vi "measure(SubVI).vi"(1 "config":refnum<queue>, 11 "error in (no error)":errorcluster) -> (4 "data":string[](array[string]), 15 "error out":errorcluster)   [LabVIEW 2019, in "SubVI.lvlib"]
uses:
  SubVI.lvlib
  config.ctl
  Instrument.ctl
  lib/QDInstrument.dll
  <vilib>/NI/Modbus Library/API/Master/Modbus Master.lvclass
  lib/Keithley 2400/Keithley 24XX/Public/Data/Read (Single Point).vi
  lib/Keithley 2400/Keithley 24XX/Keithley 24XX.lvlib
  <vilib>/measure/NI_MABase.lvlib
panel:
  # "(真是通道1，假是通道2)"
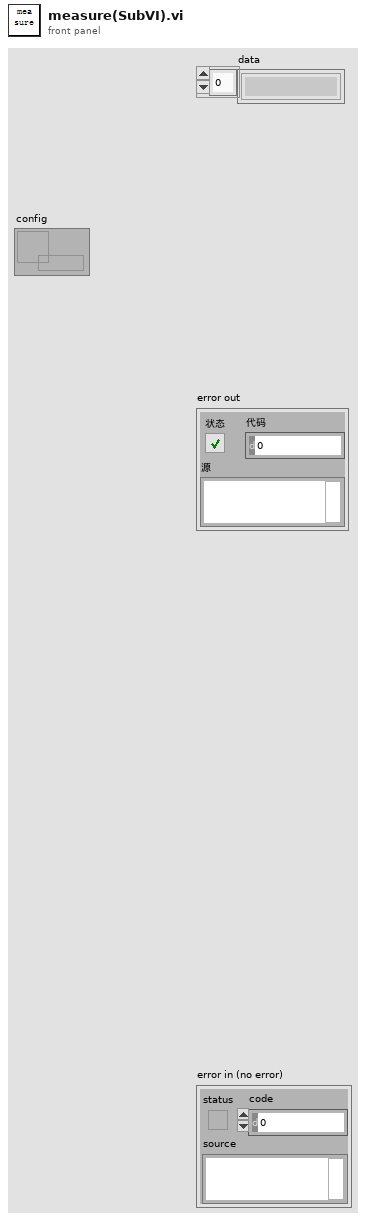
[diagram p1: front panel]
types:
  T1 = typedef "config.ctl" = cluster{"initialize":string, "6221":cluster{"6221 Resource":refnum<visa-resource-name>, "Delta status":bool}, "7001":cluster{"Ch":bool}, "SR830+6221":cluster{"source":u16, "阻抗":dbl, "量程入 4":i32, "量程入 3":i32, "量程入 2":i32, "量程入 1":i32, "电流":dbl, "SR830 2":bool, "SR830 3":bool, "SR830 4":bool, "SR830 1":bool, "VISA 1":refnum<visa-resource-name>, "VISA 2":refnum<visa-resource-name>, "VISA 3":refnum<visa-resource-name>, "VISA 4":refnum<visa-resource-name>, "量程":enum16{"量程每次测量会判定", "量程不变为设定值"}}, "2400":cluster{"2400":bool, "VISA":refnum<visa-resource-name>}, "ch":cluster{"ch str":string, "ch1":bool, "ch2":bool, "布尔":bool}, "error":bool, "数据文件路径":path, "log":cluster{"log路径":path, "log interval":dbl}, "Instrument":T2}
  T2 = typedef "Instrument.ctl" = cluster{"335 Resource":refnum<visa-resource-name>, "Input (0:A)":u16, "Instrument Type":i32, "quantum design":refnum<k24>, "Heater Output (1:1)":u16, "335state":refnum<vi>, "semaphore":T3, "TCP master instance":refnum<class "Modbus Master.lvclass">}
  T3 = typedef "Semaphore RefNum" = refnum<k1>
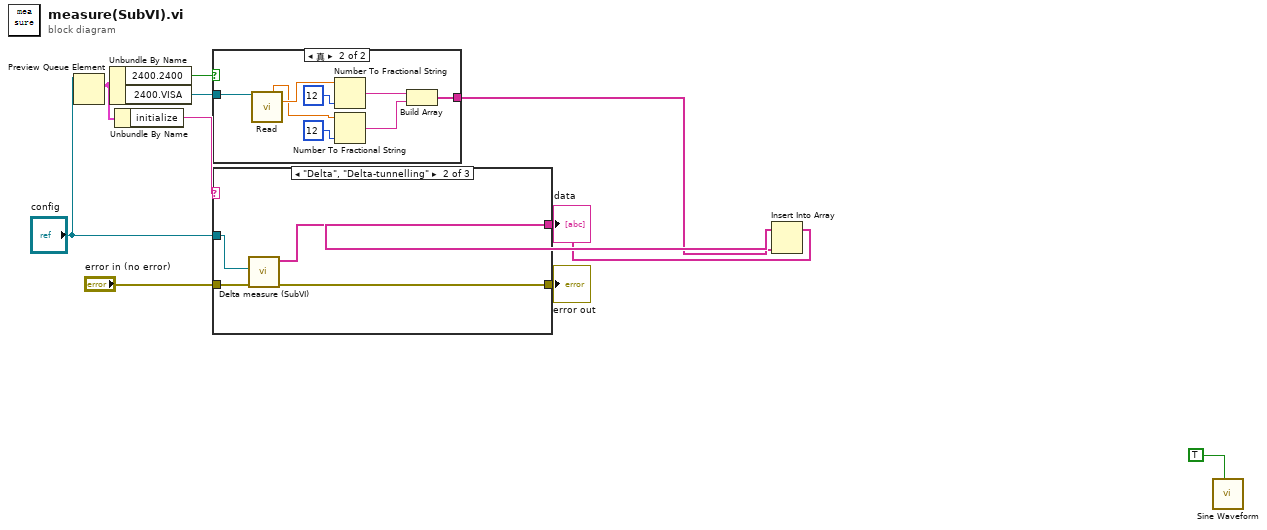
[diagram p0: block diagram]
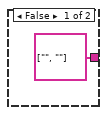
[diagram p2: hidden frame]
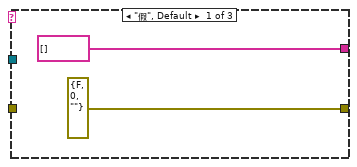
[diagram p3: hidden frame]
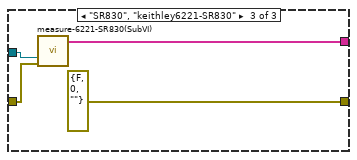
[diagram p4: hidden frame]
diagram:
  n1 = Preview Queue Element(queue="config") -> (element=w5:T1)  [unwired: 2 in, 3 out]
  n2 = Unbundle By Name(w5) -> ("2400.2400"=w7:bool, "2400.VISA"=w6:refnum<visa-resource-name>)
  n3 = Unbundle By Name(w5) -> ("initialize"=w11:string)
  n4 = case shown="真" w7 {
    tunnel: w6 -> [_ w20]
    tunnel: [string[] ["", ""] w13] -> w3
    frame False {
    }
    frame True {
      n5 = call-poly "Read.vi"("VISA resource name"=w20) -> ("Voltage"=w17:sgl, "Current"=w18:sgl)  [unwired: 8 in, 5 out]
      n6 = Number To Fractional String(number=w18, precision (6)=i16 12 ("精度(6)")) -> (F-format string=w15:string)  [unwired: 2 in]
      n7 = Number To Fractional String(number=w17, precision (6)=i16 12 ("精度(6)")) -> (F-format string=w14:string)  [unwired: 2 in]
      n8 = Build Array(w15, w14) -> (w13:string[])
    }
  }
  n9 = case shown="\"Delta\", \"Delta-tunnelling\"" w11 {
    tunnel: "config" -> [_ w26 w30]
    tunnel: [string[] [] w25 w27] -> w4
    tunnel: "error in (no error)" -> [_ w24 w29]
    tunnel: [errorcluster {"status"=FALSE, "code"=0, "source"=""} ("error out") w23 errorcluster {"status"=FALSE, "code"=0, "source"=""} ("error out")] -> w8
    frame "假", Default {
    }
    frame "Delta", "Delta-tunnelling" {
      n10 = call "Delta measure (SubVI).vi"("错误输入（无错误）"=w24, "config"=w26) -> ("错误输出"=w23:errorcluster, "数组"=w25:string[])  [unwired: 8 in]
    }
    frame "SR830", "keithley6221-SR830" {
      n11 = call "measure-6221-SR830(SubVI).vi"("config"=w30, "错误输入"=w29) -> ("输出数组"=w27:string[])  [unwired: 12 in, 1 out]
    }
  }
  "error out" <- w8
  n12 = Insert Into Array(array=w4, new element=w3) -> (→"data":string[])  [unwired: 1 in]
  n13 = call <vilib>:"Sine Waveform.vi"("reset signal"=TRUE) -> ()  [unwired: 9 in, 2 out]
